vi "HapticSTM-CurrentResponseTest.vi"() -> ()   [LabVIEW 2017]
uses:
  <vilib>/Analysis/3filter.llb/Filter Passband Type.ctl
  <vilib>/Utility/file.llb/Read Delimited Spreadsheet (DBL).vi
  Users/Brar_Lab_2/Documents/Haptic/GlobalClicksHeight.vi
  <userlib>/PositionDLL/PositionDLL.lvlib
  <vilib>/ptbypt/NI_PtbyPt.lvlib
  <vilib>/Analysis/NI_AALBase.lvlib
panel:
  out "Button":bool
  out "Zpos":cluster{dbl, "Y":dbl, i16}(graph)
  out "Filtered Current":dbl
  in  "Reset Clicks":bool
  out "Scaled Force and Current":cluster{dbl, "Filtered x":dbl, dbl}(graph)
  in  "Maximum (pA)":dbl=9000.0
  in  "Setpoint (pA)":dbl=100.0
  out "PLANE HEIGHT":dbl
  out "Current":dbl
  out "Origin Y":dbl
  out "Origin X":dbl
  out "Output Z":dbl
  in  "Rough adjust":dbl
  out "Nano Z":dbl
  out "Width":dbl
  out "VY":dbl
  out "VZ":dbl
  out "VX":dbl
  in  "Drag":dbl=1.0
  in  "STOP":bool
  in  "START":bool
  out "Fy":dbl
  out "Fz":dbl
  out "phi":dbl
  out "psi":dbl
  out "Fx":dbl
  out "theta":dbl
  out "x":dbl
  out "y":dbl
  out "z":dbl
  in  "Fine adjust":dbl=3.5
  out "Clicks":dbl
  out "Height":dbl
  # "Sample Window"
  # "Position"
  # "Sensitivity"
  # "Force"
  # "STM I/O"
  # "Angles"
  # "Current"
  # "Velocity"
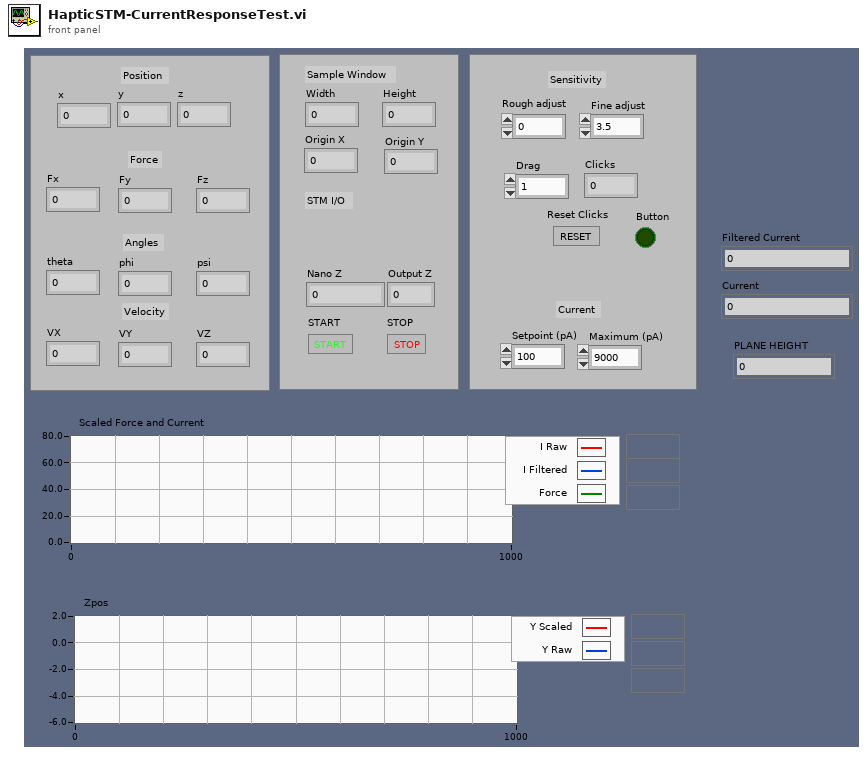
[diagram p1: front panel]
types:
  T1 = typedef "NI_AALBase.lvlib/Filter Passband Type.ctl" = enum32{"Lowpass", "Highpass", "Bandpass", "Bandstop"}
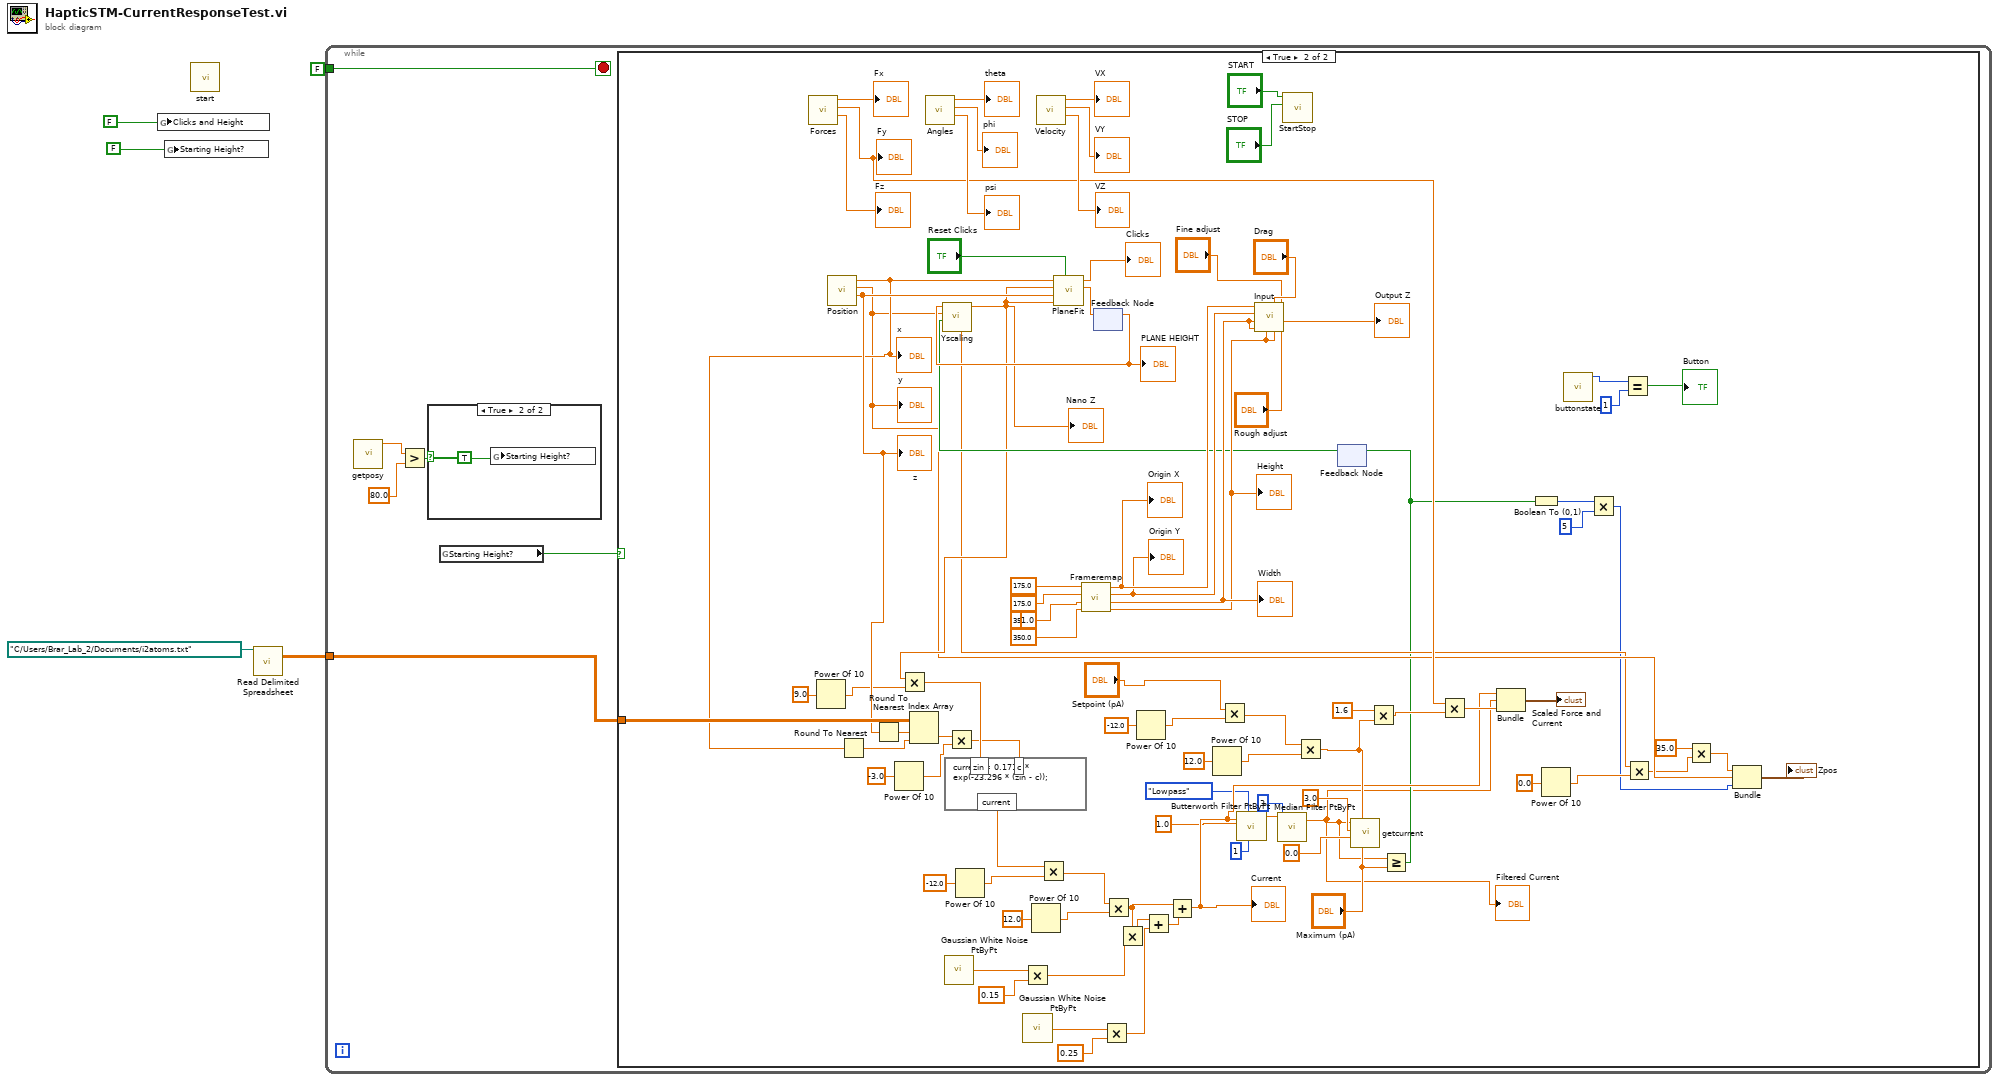
[diagram p0: block diagram]
diagram:
  n1 = global write "GlobalClicksHeight.vi" "Clicks and Height"(FALSE ("Clicks and Height")) -> ()
  n2 = global write "GlobalClicksHeight.vi" "Starting Height?"(FALSE ("Clicks and Height")) -> ()
  n3 = call <userlib>:"start.vi"() -> ()  [unwired: 11 in, 1 out]
  n4 = call-poly <vilib>:"Read Delimited Spreadsheet.vi"("file path (dialog if empty)"=path "C:/Users/Brar_Lab_2/Documents/i2atoms.txt") -> ("all rows"=w4:dbl[][])  [unwired: 9 in, 5 out]
  n5 = while {
    tunnel: FALSE -> [w11]
    tunnel: w4 -> [w10]
    stop <- w11 stop-if-true
    n6 = call <userlib>:"getposy.vi"() -> ("function return"=w9:dbl)  [unwired: 11 in]
    n7 = Greater?(x=w9, y=80.0) -> (0:w7:bool)
    n8 = case shown="True" w7 {
      frame False {
      }
      frame True {
        n9 = global write "GlobalClicksHeight.vi" "Starting Height?"(TRUE ("Clicks and Height")) -> ()
      }
    }
    n10 = global read "GlobalClicksHeight.vi" "Starting Height?"() -> (w6:bool)
    n11 = case shown="True" w6 {
      tunnel: w10 -> [_ w64]
      frame False {
      }
      frame True {
        (unwired) 1.0 ("FO X")
        n12 = call <userlib>:"Forces.vi"() -> ("Fz"=→"Fz":dbl, "Fy"=w50:dbl, "Fx"=→"Fx":dbl)  [unwired: 9 in]
        "Fy" <- w50
        n13 = Power Of 10(x=9.0) -> (10^x=w58:dbl)
        n14 = call <userlib>:"Position.vi"() -> ("Z"=w61:dbl, "Y"=w31:dbl, "X"=w60:dbl)  [unwired: 9 in]
        "x" <- w60
        "y" <- w31
        "z" <- w61
        n15 = Round To Nearest(number=w60) -> (nearest integer value=w62:dbl)
        n16 = Round To Nearest(number=w61) -> (nearest integer value=w63:dbl)
        n17 = Power Of 10(x=-3.0) -> (10^x=w53:dbl)
        n18 = Index Array(array=w64, index (row)=w63, index (col)=w62) -> (element=w54:dbl)
        n19 = call <userlib>:"Angles.vi"() -> ("psi"=→"psi":dbl, "phi"=→"phi":dbl, "theta"=→"theta":dbl)  [unwired: 9 in]
        n20 = call <vilib>:"Gaussian White Noise PtByPt.vi"() -> ("Gaussian white noise"=w49:dbl)  [unwired: 3 in]
        n21 = Multiply(x=w54, y=w53) -> (x*y=w52:dbl)
        n22 = Power Of 10(x=-12.0) -> (10^x=w75:dbl)
        n23 = Multiply(x=w49, y=0.15) -> (x*y=w47:dbl)
        n24 = call <vilib>:"Gaussian White Noise PtByPt.vi"() -> ("Gaussian white noise"=w44:dbl)  [unwired: 3 in]
        n25 = Power Of 10(x=12.0) -> (10^x=w84:dbl)
        n26 = call <userlib>:"Velocity.vi"() -> ("VZ"=→"VZ":dbl, "VY"=→"VY":dbl, "VX"=→"VX":dbl)  [unwired: 9 in]
        n27 = call <userlib>:"Frameremap.vi"("FH"=350.0 ("FO X"), "FW"=350.0 ("FO X"), "FO Z"=175.0 ("FO X"), "FO X"=175.0) -> ("FH"=w91:dbl, "FW"=w92:dbl, "Z Origin"=w76:dbl, "X Origin"=w77:dbl)  [unwired: 4 in]
        "Height" <- w91
        "Width" <- w92
        "Origin X" <- w77
        "Origin Y" <- w76
        n28 = feedback #1() -> (w78:dbl)  [unwired: 1 in]
        "PLANE HEIGHT" <- w78
        n29 = Multiply(x=w44, y=0.25) -> (x*y=w40:dbl)
        n30 = Power Of 10(x=-12.0) -> (10^x=w70:dbl)
        n31 = Power Of 10(x=12.0) -> (10^x=w72:dbl)
        n32 = Multiply(x="Setpoint (pA)", y=w70) -> (x*y=w68:dbl)
        n33 = call <userlib>:"Input.vi"("Current * 10^input"="Rough adjust", "Sensitivity"="Fine adjust", "Scopez"=w91, "Drag"="Drag", "FH"=w91, "FW"=w92, "Scopex"=w92, "Z origin"=w76, "X origin"=w77) -> ("Scaled Current"=→"Output Z":dbl)  [unwired: 2 in]
        n34 = call <userlib>:"StartStop.vi"("STOP"="STOP", "START"="START") -> ()  [unwired: 10 in]
        n35 = Multiply(x=w68, y=w72) -> (x*y=w37:dbl)
        n36 = feedback #2() -> (w66:bool)  [unwired: 1 in]
        n37 = call <userlib>:"Yscaling.vi"("Current Maxed?"=w66, "Y"=w31, "Plane Height"=w78) -> ("y scaled"=w33:dbl, "Testoutput"=w27:dbl)  [unwired: 7 in]
        "Nano Z" <- w33
        n38 = Multiply(x=w33, y=w58) -> (x*y=w56:dbl)
        n39 = formula code="current = 0.1714 * exp(-23.296 * (zin - c));"("zin"=w56, "c"=w52) -> ("current"=w59:dbl)
        n40 = Multiply(x=w59, y=w75) -> (x*y=w73:dbl)
        n41 = call <userlib>:"PlaneFit.vi"("Reset Clicks"="Reset Clicks", "Y PEN"=w33, "Z"=w61, "Nano Z"=w33, "X"=w60) -> ("Output"=w87:dbl, "Clicks"=→"Clicks":dbl)  [unwired: 5 in]
        n42 = feedback-in #1(w87) -> ()
        n43 = Multiply(x=w73, y=w84) -> (x*y=w46:dbl)
        n44 = Multiply(x=w46, y=w47) -> (x*y=w41:dbl)
        n45 = Add(x=w41, y=w40) -> (x+y=w42:dbl)
        n46 = Add(x=w46, y=w42) -> (x+y=w23:dbl)
        "Current" <- w23
        n47 = call <vilib>:"Butterworth Filter PtByPt.vi"("order"=1, "filter type"=Filter_Passband_Type."Lowpass", "sampling freq: fs"=1.0, "x"=w23) -> ("Filtered x"=w15:dbl)  [unwired: 5 in, 1 out]
        n48 = call <vilib>:"Median Filter PtByPt.vi"("rank"=3, "x"=w15) -> ("Filtered x"=w14:dbl)  [unwired: 2 in, 1 out]
        "Filtered Current" <- w14
        n49 = call <userlib>:"getcurrent.vi"("maxcurrentin"="Maximum (pA)", "setpoint"=w37, "minforcey"=0.0, "maxforcey"=3.0, "currentin"=w14) -> ()  [unwired: 7 in]
        n50 = Multiply(x=1.6 ("y"), y=w37) -> (x*y=w38:dbl)
        n51 = Greater Or Equal?(x=w14, y="Maximum (pA)") -> (x >= y?=w20:bool)
        n52 = feedback-in #2(w20) -> ()
        n53 = Multiply(x=w50, y=w38) -> (x*y=w45:dbl)
        n54 = Bundle(w23, "Filtered x"=w14, w45) -> (→"Scaled Force and Current":cluster{dbl, "Filtered x":dbl, dbl})  [unwired: 1 in]
        n55 = Boolean To (0,1)(Boolean=w20) -> (0, 1=w19:i16)
        n56 = Power Of 10(x=0.0) -> (10^x=w35:dbl)
        n57 = call <userlib>:"buttonstate.vi"() -> ("function return"=w26:i32)  [unwired: 11 in]
        n58 = Multiply(x=w19, y=i16 5) -> (x*y=w17:i16)
        n59 = Equal?(x=w26, y=1) -> (x = y?=→"Button":bool)
        n60 = Multiply(x=w27, y=w35) -> (x*y=w29:dbl)
        n61 = Multiply(x=35.0, y=w29) -> (x*y=w30:dbl)
        n62 = Bundle(w30, "Y"=w31, w17) -> (→"Zpos":cluster{dbl, "Y":dbl, i16})  [unwired: 1 in]
      }
    }
  }
